vi "sound_gen.vi"(0 "tones":T1(array[cluster])=[{"frequency"=10.0, "amplitude"=1.0, "phase"=0.0}, {"frequency"=20.0, "amplitude"=0.1, "phase"=0.0}] {"phase" format="%.2p"; "amplitude" format="%0.2p"; "frequency" format="%0.2p"}, 5 "sampling info":cluster{"Fs":dbl, "#s":dbl}={"Fs"=10000.0, "#s"=200.0} {"Fs" format="%.2p"}, 7 "Boolean":bool, 9 "tones 2":T1(array[cluster])=[{"frequency"=10.0, "amplitude"=1.0, "phase"=0.0}, {"frequency"=20.0, "amplitude"=0.1, "phase"=0.0}] {"phase" format="%.2p"; "amplitude" format="%0.2p"; "frequency" format="%0.2p"}, 11 "sampling info 2":cluster{"Fs":dbl, "#s":dbl}={"Fs"=10000.0, "#s"=600.0} {"Fs" format="%.2p"}) -> (6 "signal out":waveform(dbl)(graph))   [LabVIEW 2022 SP3]
uses:
  <vilib>/measure/NI_MABase.lvlib
panel:
  out "error out":errorcluster
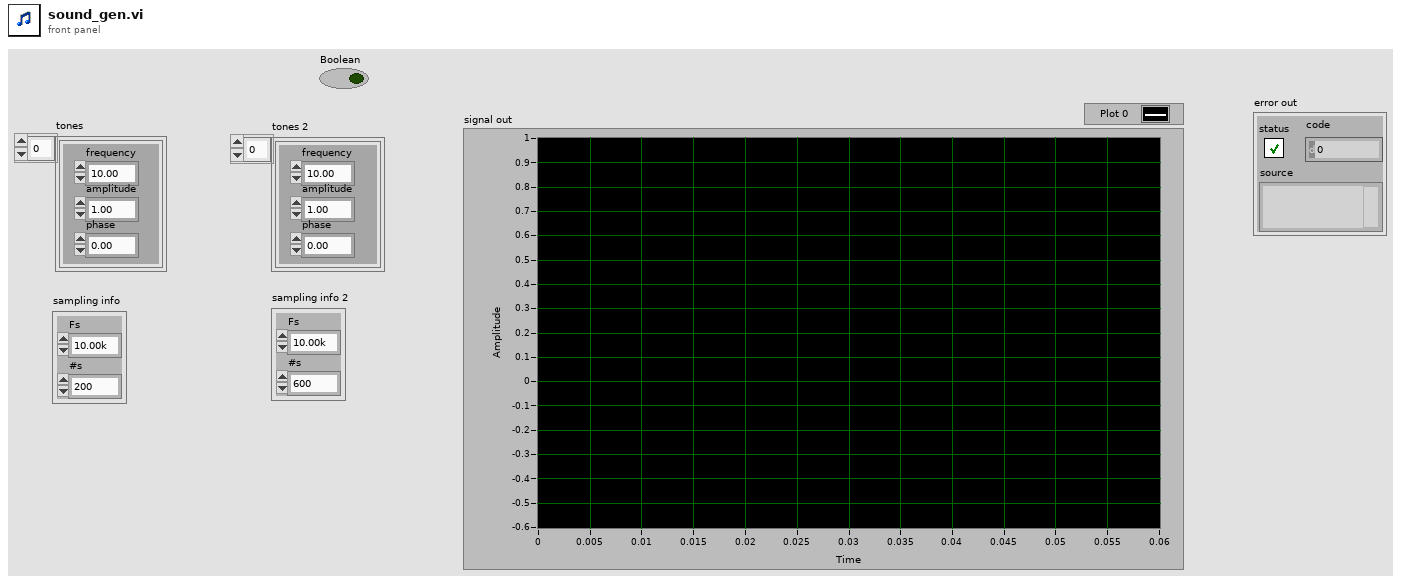
[diagram p1: front panel]
types:
  T1 = cluster{"frequency":dbl, "amplitude":dbl, "phase":dbl}[]
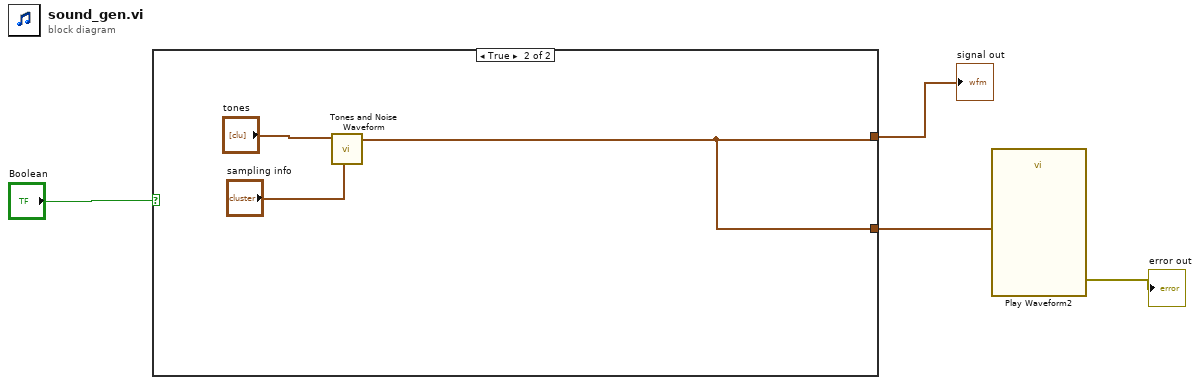
[diagram p0: block diagram]
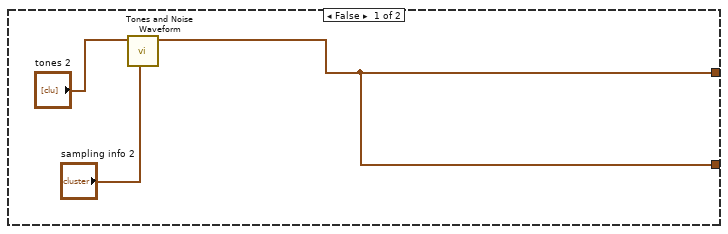
[diagram p2: hidden frame]
diagram:
  n1 = case shown="True" "Boolean" {
    tunnel: [w5 w8] -> w2
    tunnel: [w5 w8] -> w1
    frame False {
      n2 = call <vilib>:"Tones and Noise Waveform.vi"("sampling info"="sampling info 2", "tones"="tones 2") -> ("signal out"=w5:waveform(dbl))  [unwired: 8 in, 1 out]
    }
    frame True {
      n3 = call <vilib>:"Tones and Noise Waveform.vi"("sampling info"="sampling info", "tones"="tones") -> ("signal out"=w8:waveform(dbl))  [unwired: 8 in, 1 out]
    }
  }
  "signal out" <- w1
  n4 = call "Play Waveform2"("Data"=w2) -> ("error out"=→"error out":errorcluster)  [unwired: 18 in]
